vi "HMAC.vi"(10 "Key":string, 11 "Message":string) -> (3 "Keyed Hash":string)   [LabVIEW 2015, in "NI_AWS Core.lvlib"]
uses:
  NI_AWS Core.lvlib
  <vilib>/LVH/i3 External Encryption/i3-external-encryption.lvlib
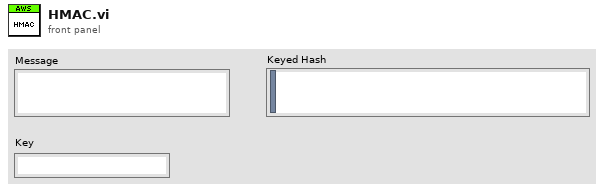
[diagram p1: front panel]
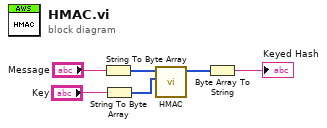
[diagram p0: block diagram]
diagram:
  n1 = String To Byte Array(string="Message") -> (unsigned byte array=w5:u8[])
  n2 = String To Byte Array(string="Key") -> (unsigned byte array=w4:u8[])
  n3 = call <vilib>:"HMAC.vi"("Key"=w4, "Message"=w5) -> ("HMAC digest"=w2:u8[])  [unwired: 7 in, 2 out]
  n4 = Byte Array To String(unsigned byte array=w2) -> (string=→"Keyed Hash":string)
